vi "BaslangicKapanmaKontrol.vi"(10 "Normal Kapanma":bool, 11 "queue":refnum<queue>) -> ()   [LabVIEW 2021]
panel:
  out "Durum":string
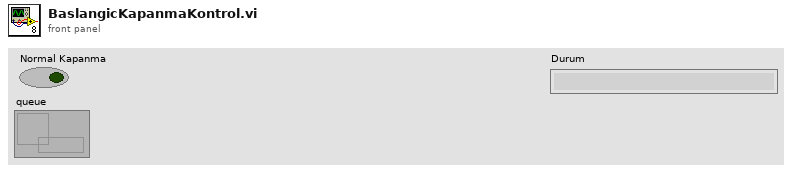
[diagram p1: front panel]
types:
  T1 = cluster{"element":string, "Message Data":variant}
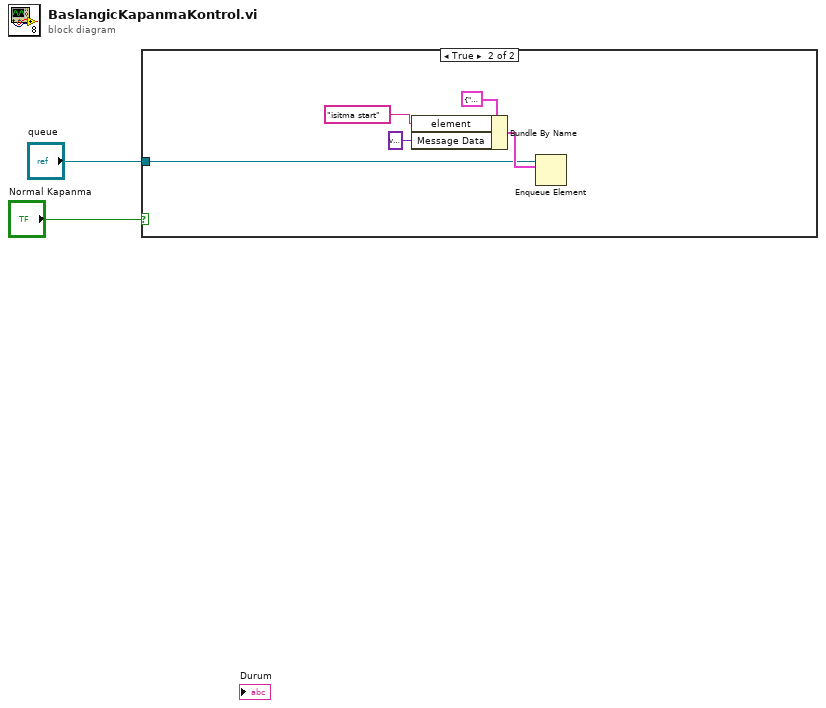
[diagram p0: block diagram]
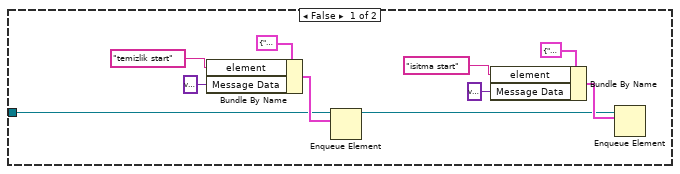
[diagram p2: hidden frame]
diagram:
  n1 = case shown="True" "Normal Kapanma" {
    tunnel: "queue" -> [w4 w14]
    frame False {
      n2 = Bundle By Name(cluster=T1 {"element"="", "Message Data"=variant}, "element"="temizlik start", "Message Data"=variant) -> (w5:T1)
      n3 = Enqueue Element(queue=w4, element=w5) -> (queue out=w3:refnum<queue>)  [unwired: 2 in, 2 out]
      n4 = Bundle By Name(cluster=T1 {"element"="", "Message Data"=variant}, "element"="isitma start", "Message Data"=variant) -> (w12:T1)
      n5 = Enqueue Element(queue=w3, element=w12) -> ()  [unwired: 2 in, 3 out]
    }
    frame True {
      n6 = Bundle By Name(cluster=T1 {"element"="", "Message Data"=variant}, "element"="isitma start", "Message Data"=variant) -> (w17:T1)
      n7 = Enqueue Element(queue=w14, element=w17) -> ()  [unwired: 2 in, 3 out]
    }
  }
